vi "onlineanalysis.vi"() -> ()   [LabVIEW 2010]
uses:
  Fear Conditioning/GlobalFear.vi
panel:
  out "HR":dbl
  out "Waveform Chart":i32[](graph)
  in  "stop":bool
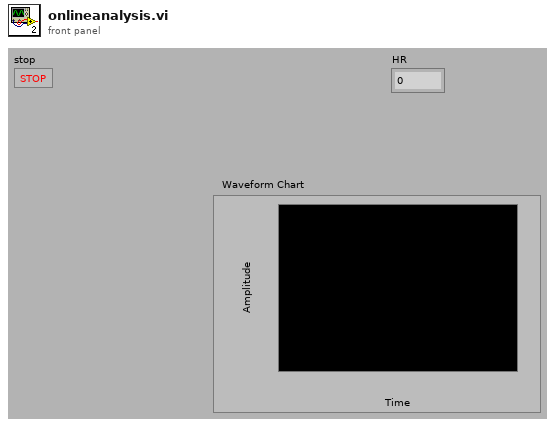
[diagram p1: front panel]
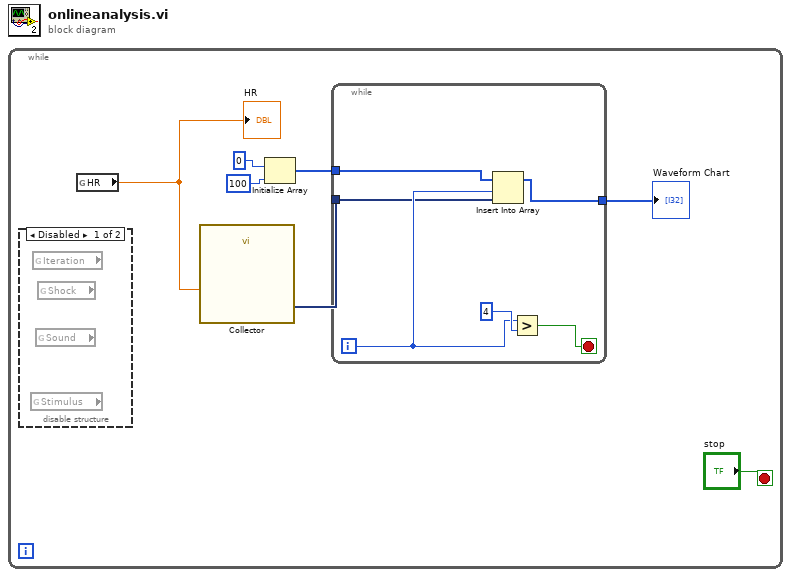
[diagram p0: block diagram]
diagram:
  n1 = while {
    stop <- "stop" stop-if-true
    n2 = disable-structure shown="Disabled" {
      frame Disabled {
        n3 = global read "GlobalFear.vi" "Stimulus"() -> ()  [unwired: 1 out]
        n4 = global read "GlobalFear.vi" "Iteration"() -> ()  [unwired: 1 out]
        n5 = global read "GlobalFear.vi" "Sound"() -> ()  [unwired: 1 out]
        n6 = global read "GlobalFear.vi" "Shock"() -> ()  [unwired: 1 out]
      }
      frame Enabled {
      }
    }
    n7 = global read "GlobalFear.vi" "HR"() -> (w5:dbl)
    "HR" <- w5
    n8 = call "Collector"("Signals"=w5) -> ("Collected Signals"=w4:dynamicdata)  [unwired: 9 in, 1 out]
    n9 = Initialize Array(0, 100) -> (w1:i32[])
    n10 = while {
      tunnel: [w13] -> w6
      tunnel: w4 -> [w9]
      tunnel: w1 -> [w8]
      i -> [w10]
      stop <- w11 stop-if-true
      n11 = Insert Into Array(array=w8, index=w10, new element=w9) -> (w13:i32[])
      n12 = Greater?(x=w10, y=4) -> (0:w11:bool)
    }
    "Waveform Chart" <- w6
  }
